vi "MakeRunList.vi"(7 "error in":errorcluster, 10 "WheelList":string[][](array[string])) -> (0 "error out":errorcluster, 1 "Runlist":i32[](array[numeric]), 2 "SampleCount":i32, 3 "First Sample":i32)   [LabVIEW 2013]
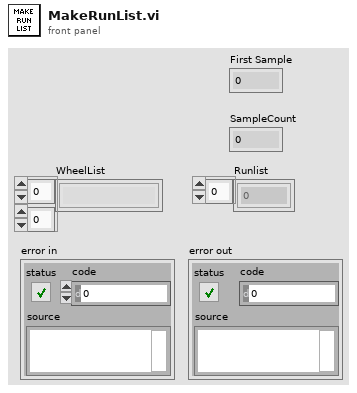
[diagram p1: front panel]
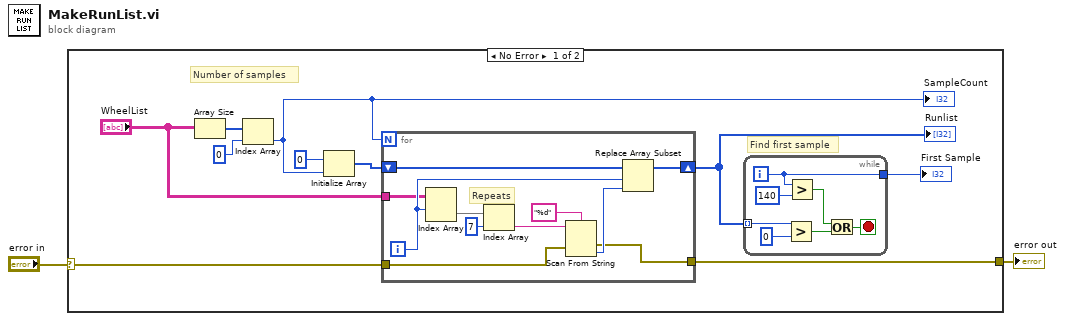
[diagram p0: block diagram]
diagram:
  n1 = case shown="No Error" "error in" {
    selector: "error in" -> [w6 w31]
    tunnel: [w5 w31] -> w1
    frame No Error {
      # "Find first sample"
      # "Number of samples"
      n2 = Array Size(array="WheelList") -> (size(s)=w12:i32[])
      n3 = Index Array(array=w12, index=0) -> (element=w8:i32)
      "SampleCount" <- w8
      n4 = Initialize Array(0 ("element"), w8) -> (w9:i32[])
      n5 = for {
        N: w8 -> [_]
        shift-right: [w30] -> w3
        shift-left: w9 -> [w23]
        tunnel: "WheelList" -> [w22]
        tunnel: w6 -> [w21]
        tunnel: [w20] -> w5
        i -> [w25]
        # "Repeats"
        n6 = Index Array(array=w22, index (row)=w25) -> (element=w24:string[])  [unwired: 1 in]
        n7 = Index Array(array=w24, index=7) -> (element=w28:string)
        n8 = Scan From String(format string="%d", input string=w28, error in=w21) -> (error out=w20:errorcluster, output 1=w26:i32)  [unwired: 1 in, 3 out]
        n9 = Replace Array Subset(array=w23, new element=w26, index=w25) -> (w30:i32[])
      }
      "Runlist" <- w3
      n10 = while {
        tunnel: w3 -> [w17] mode=indexing
        tunnel: [w15] -> w4
        i -> [w15]
        stop <- w16 stop-if-true
        n11 = Greater?(x=w17, y=0) -> (0:w18:bool)
        n12 = Greater?(x=w15, y=140) -> (0:w13:bool)
        n13 = Or(x=w13, y=w18) -> (x .or. y?=w16:bool)
      }
      "First Sample" <- w4
    }
    frame Error {
    }
  }
  "error out" <- w1
